vi "Cross_spectra_and_phase.vi"(0 "U1":dbl[](array[numeric]) format="%.2f", 2 "U2":dbl[](array[numeric]) format="%.2f") -> (5 "U1 spectra":cluster{dbl, dbl, dbl[]}(graph), 6 "U2 spectra":cluster{dbl, dbl, dbl[]}(graph), 7 "U1 U2 coherence":cluster{dbl, dbl, "Coherence array":dbl[]}(graph), 8 "U1 U2 phase":cluster{dbl, dbl, "Phase array":dbl[]}(graph))   [LabVIEW 2011]
uses:
  Globals/Meas_global.vi
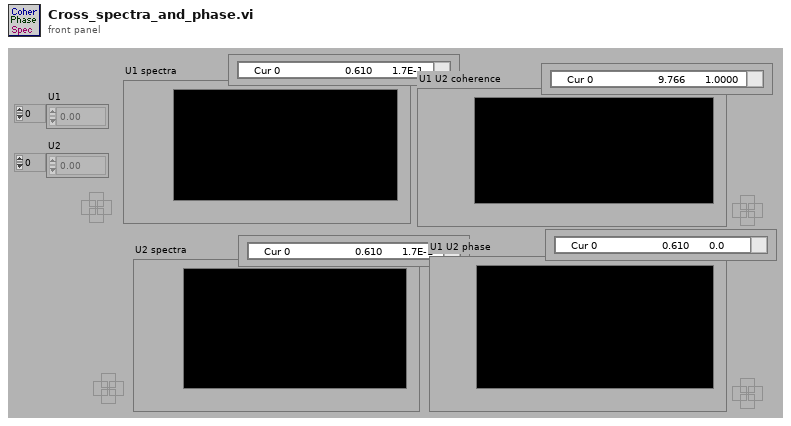
[diagram p1: front panel]
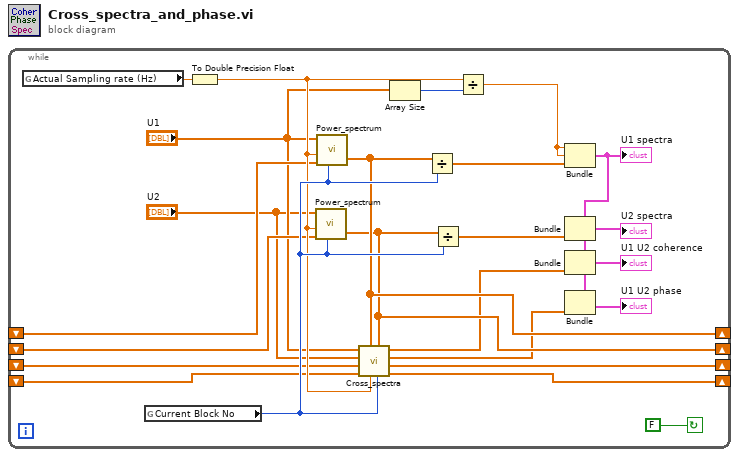
[diagram p0: block diagram]
diagram:
  n1 = while {
    shift-left: _ -> [w19]
    shift-right: [w17] -> _
    shift-left: _ -> [w20]
    shift-right: [w18] -> _
    shift-left: _ -> [w21]
    shift-right: [w15] -> _
    shift-left: _ -> [w22]
    shift-right: [w16] -> _
    stop <- FALSE continue-if-true
    n2 = global read "Meas_global.vi" "Actual Sampling rate (Hz)"() -> (w5:dbl)
    n3 = global read "Meas_global.vi" "Current Block No"() -> (w24:i32)
    n4 = To Double Precision Float(number=w5) -> (double precision float=w23:dbl)
    n5 = call "Power_spectrum.vi"("U"="U2", "Sampling frequency"=w23, "Spectrum input array"=w21, "Block No"=w24) -> ("Spectrum output array"=w15:dbl[])  [unwired: 1 in, 1 out]
    n6 = call "Power_spectrum.vi"("U"="U1", "Sampling frequency"=w23, "Spectrum input array"=w22, "Block No"=w24) -> ("Spectrum output array"=w16:dbl[])  [unwired: 1 in, 1 out]
    n7 = call "Cross_spectra.vi"("block number"=w24, "S11 input array"=w15, "sampling frequency"=w23, "S22 input array"=w16, "Im(S12) input array"=w19, "Re(S12) input array"=w20, "U2"="U2", "U1"="U1") -> ("Im(S12) output array"=w17:dbl[], "Re(S12) output array"=w18:dbl[], "Phase array"=w10:dbl[], "Coherence array"=w11:dbl[])
    n8 = Array Size(array="U1") -> (size(s)=w9:i32)
    n9 = Divide(x=w16, y=w24) -> (x/y=w13:dbl[])
    n10 = Divide(x=w15, y=w24) -> (x/y=w12:dbl[])
    n11 = Divide(x=w23, y=w9) -> (x/y=w3:dbl)
    n12 = Bundle(w3, w3, w13) -> (w4:cluster{dbl, dbl, dbl[]})  [unwired: 1 out]
    "U1 spectra" <- w4
    n13 = Bundle(cluster=w4, w12) -> (→"U2 spectra":cluster{dbl, dbl, dbl[]})  [unwired: 2 out]
    n14 = Bundle(cluster=w4, w11) -> (→"U1 U2 coherence":cluster{dbl, dbl, dbl[]})  [unwired: 2 out]
    n15 = Bundle(cluster=w4, w10) -> (→"U1 U2 phase":cluster{dbl, dbl, dbl[]})  [unwired: 2 out]
  }
